vi "20SimModelCalculateStep.vi"(7 "OutputArrayInitial":dbl[](array[numeric]), 9 "time in":dbl, 10 "InputArray":dbl[](array[numeric])) -> (1 "OutputArray":dbl[](array[numeric]), 2 "time out":dbl, 3 "ReturnValue":i32)   [LabVIEW 2011]
uses:
  lv20simmodel.dll
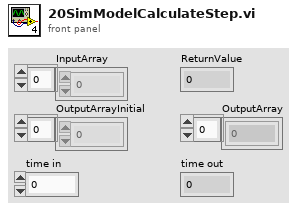
[diagram p1: front panel]
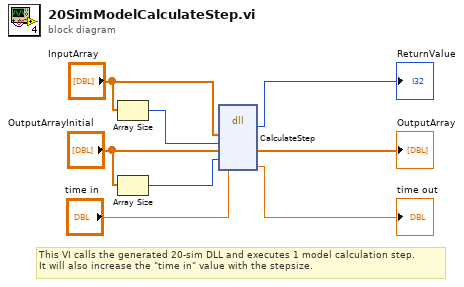
[diagram p0: block diagram]
diagram:
  # "This VI calls the generated 20-sim DLL and executes 1 model calculation step.\nIt will also increase the \"time in\" value with the stepsize."
  n1 = Array Size(array="InputArray") -> (size(s)=w4:i32)
  n2 = Array Size(array="OutputArrayInitial") -> (size(s)=w2:i32)
  n3 = dll-call lib="C:/Temp/BondGraphModel/lv20simmodel.dll" fn="CalculateStep"("inarr"="InputArray", "inputs"=w4, "outarr"="OutputArrayInitial", "outputs"=w2, "time"="time in") -> ("return"=→"ReturnValue":i32, "outarr"=→"OutputArray":dbl[], "time"=→"time out":dbl)  [unwired: 6 in, 2 out]
